vi "myRIO_BRig_RT_comm_webdav_connect.vi"(10 "input_password":string, 11 "input_username":string="Paul Jonak") -> (0 "output_code":u8, 2 "output_Iconnected":bool, 3 "output_hSession":T1)   [LabVIEW 2014]
uses:
  <vilib>/WebDAVClient/Advanced/SessionHandle.ctl
  <vilib>/WebDAVClient/NI_WebDAV.lvlib
panel:
  out "error out":errorcluster
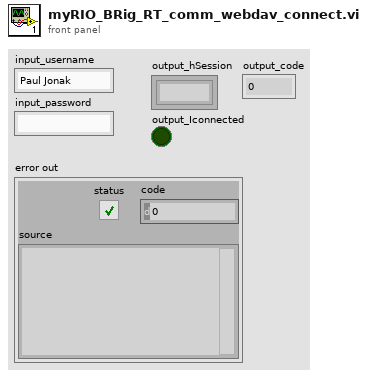
[diagram p1: front panel]
types:
  T1 = typedef "NI_WebDAV.lvlib/SessionHandle.ctl" = refnum<k1>
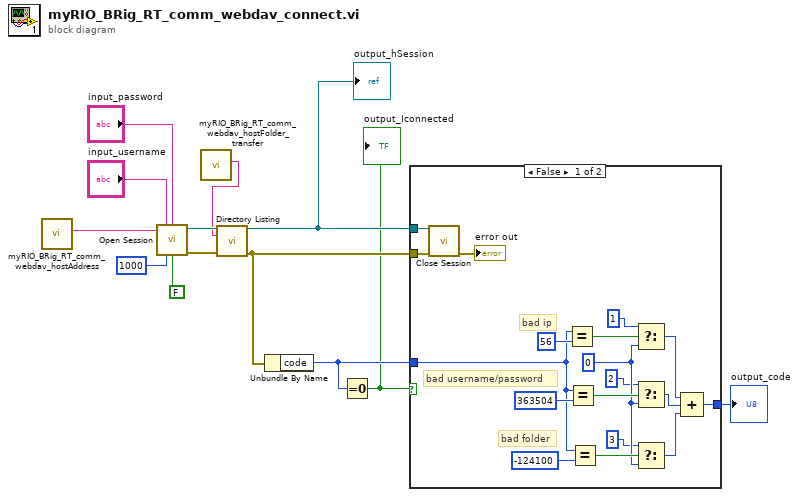
[diagram p0: block diagram]
diagram:
  n1 = call "myRIO_BRig_RT_comm_webdav_hostAddress.vi"() -> ("output_HostAddress"=w1:string)  [unwired: 11 in]
  n2 = call <vilib>:"Open Session.vi"("host uri prefix"=w1, "username"="input_username", "password"="input_password", "timeout ms"=1000, "verify server?"=FALSE) -> ("session handle out"=w12:T1, "error out"=w3:errorcluster)  [unwired: 9 in]
  n3 = call "myRIO_BRig_RT_comm_webdav_hostFolder_transfer.vi"() -> ("output_HostFolder"=w2:string)  [unwired: 11 in]
  n4 = call <vilib>:"Directory Listing.vi"("session handle"=w12, "relative uri"=w2, "error in (no error)"=w3) -> ("session handle out"=w9:T1, "error out"=w8:errorcluster)  [unwired: 9 in, 2 out]
  "output_hSession" <- w9
  n5 = Unbundle By Name(w8) -> ("code"=w6:i32)
  n6 = Equal To 0?(x=w6) -> (x = 0?=w5:bool)
  "output_Iconnected" <- w5
  n7 = case shown="False" w5 {
    tunnel: w6 -> [w25 _]
    tunnel: w9 -> [w30 _]
    tunnel: w8 -> [w29 _]
    tunnel: [w15 _] -> w7
    frame False {
      w21 = u8 0
      # "bad folder"
      # "bad username/password"
      # "bad ip"
      n8 = call <vilib>:"Close Session.vi"("session handle"=w30, "error in (no error)"=w29) -> ("error out"=→"error out":errorcluster)  [unwired: 13 in]
      n9 = Equal?(x=w25, y=56) -> (x = y?=w24:bool)
      n10 = Equal?(x=w25, y=363504) -> (x = y?=w23:bool)
      n11 = Equal?(x=w25, y=-124100) -> (x = y?=w22:bool)
      n12 = Select(t=u8 1, s=w24, f=w21) -> (s? t:f=w14:u8)
      n13 = Select(t=u8 2, s=w23, f=w21) -> (s? t:f=w17:u8)
      n14 = Select(t=u8 3, s=w22, f=w21) -> (s? t:f=w16:u8)
      n15 = Compound Arithmetic op=ADD(w14, w17, w16) -> (w15:u8)
    }
    frame True {
    }
  }
  "output_code" <- w7
